vi "GetMenuTagList.vi"(7 "Seperator(\"\\\")":string="\\", 8 "error in (no error) 2":errorcluster, 10 "item tag":string, 11 "menu reference":refnum<k9>) -> (0 "error in (no error)":errorcluster, 1 "Tree":string[][](array[string]), 2 "submenu tags":string[](array[string]), 3 "menu reference out":refnum<k9>)   [LabVIEW 2014]
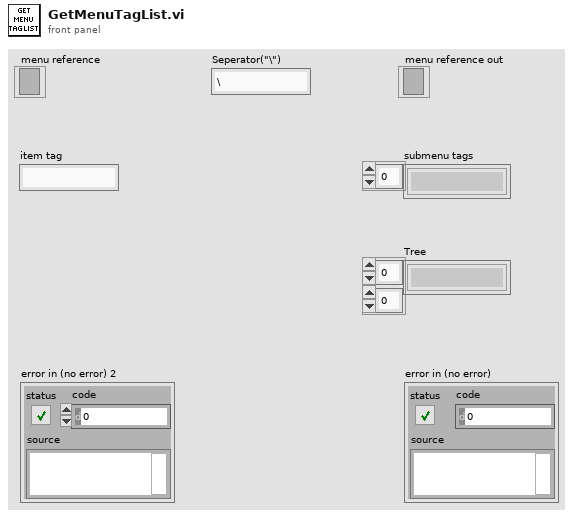
[diagram p1: front panel]
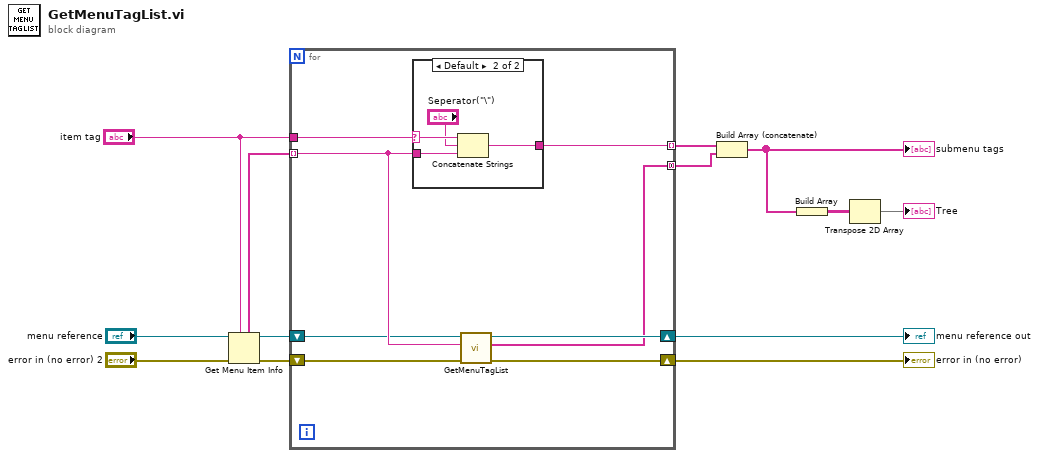
[diagram p0: block diagram]
diagram:
  n1 = Get Menu Item Info(7:"item tag", 8:"error in (no error) 2", 11:"menu reference") -> (0:w6:errorcluster, 3:w9:refnum<k9>, 5:w11:string[])  [unwired: 4 out]
  n2 = for {
    tunnel: "item tag" -> [w21]
    tunnel: w11 -> [w18] mode=indexing
    tunnel: [w14] -> w10 mode=indexing
    shift-right: [w20] -> w8
    shift-left: w9 -> [w16]
    shift-right: [w19] -> w5
    shift-left: w6 -> [w15]
    tunnel: [w17] -> w4 mode=concatenating
    n3 = case shown="Default" w21 {
      selector: w21 -> [_ w26]
      tunnel: [w22 w24] -> w14
      tunnel: w18 -> [w22 w23]
      frame "" {
      }
      frame Default {
        n4 = Concatenate Strings(w26, "Seperator(\"\\\")", w23) -> (w24:string)
      }
    }
    n5 = call "GetMenuTagList.vi"("error in (no error) 2"=w15, "item tag"=w18, "menu reference"=w16) -> ("error in (no error)"=w19:errorcluster, "submenu tags"=w17:string[], "menu reference out"=w20:refnum<k9>)  [unwired: 5 in, 1 out]
  }
  "menu reference out" <- w8
  "error in (no error)" <- w5
  n6 = Build Array (concatenate)(w10, w4) -> (w3:string[])
  "submenu tags" <- w3
  n7 = Build Array(w3) -> (w2:string[][])
  n8 = Transpose 2D Array(2D array=w2) -> (transposed array=→"Tree":string[][])
